vi "MDPtr Unpack WaveformArr.vi"(10 "error in (no error)":errorcluster, 11 "HexStrPtr":T1) -> (1 "String Attribute":string, 2 "error out":errorcluster, 3 "Waveforms":waveform(dbl)[](array[waveform]))   [LabVIEW 2017, in "MDPtr.lvlib"]
uses:
  MDPtr.lvlib
  MDPtr TypeDef/MDPtr.ctl
  MDPtr TypeDef/MDPtr SupportedDataTypeDef.ctl
  MDPtr TypeDef/MDPtr DataFrame-WaveformArr.ctl
  MDPtr TypeDef/MDPtr DataFrame-Common.ctl
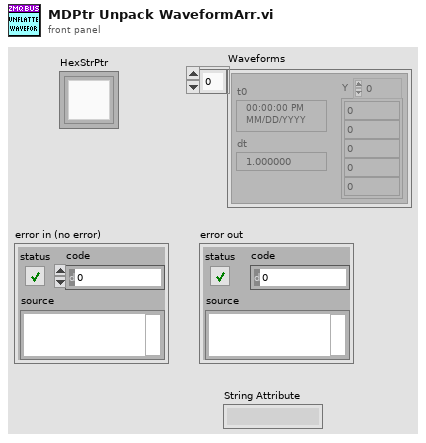
[diagram p1: front panel]
types:
  T1 = typedef "MDPtr.lvlib/MDPtr.ctl" = refnum<k1>
  T2 = typedef "MDPtr.lvlib/MDPtr SupportedDataTypeDef.ctl" = enum16{"<Invalid>", "<User 0>", "<User 1>", "<User 2>", "<User 3>", "<User 4>", "Memory", "Waveform", "Waveform Arr", "Double Arr", "String Arr"}
  T3 = typedef "MDPtr.lvlib/MDPtr DataFrame-WaveformArr.ctl" = cluster{"Common":T4, "DVR":refnum<data-value>}
  T4 = typedef "MDPtr.lvlib/MDPtr DataFrame-Common.ctl" = cluster{"Data Type":T2, "Copy Count":i32, "String Attribute":string}
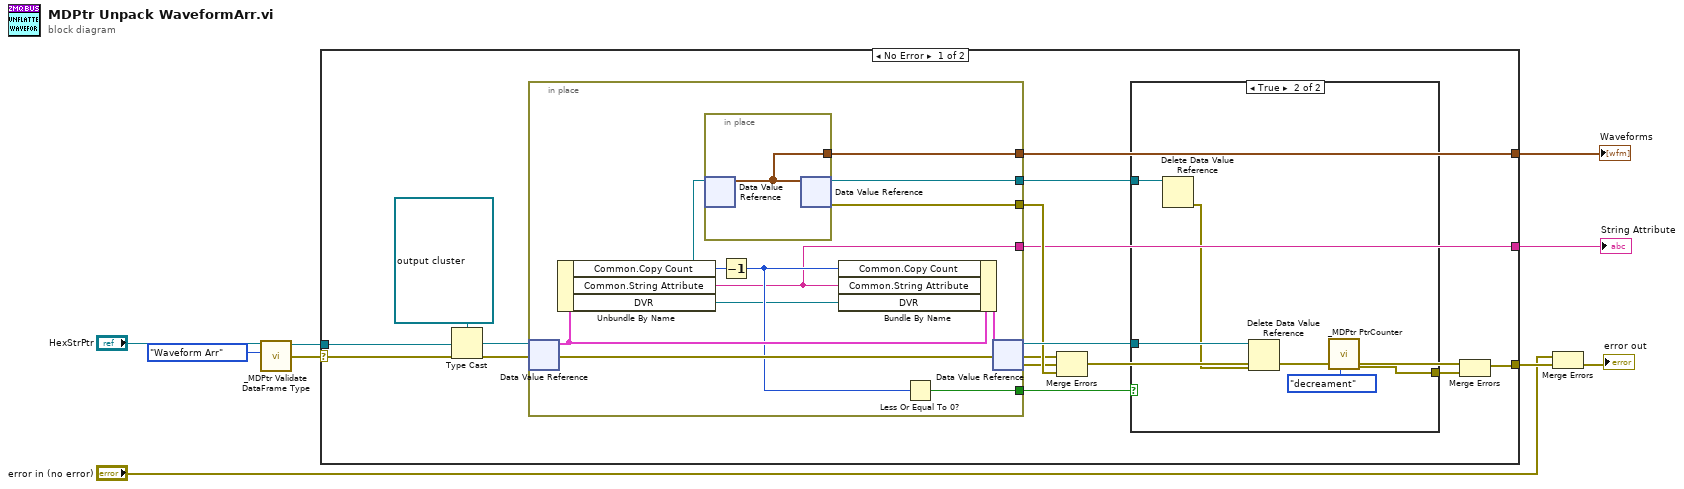
[diagram p0: block diagram]
diagram:
  n1 = call "_MDPtr Validate DataFrame Type.vi"("Data Type"=MDPtr_SupportedDataTypeDef."Waveform Arr", "data"="HexStrPtr") -> ("error out"=w2:errorcluster, "data (dup)"=w3:T1)  [unwired: 7 in]
  n2 = case shown="No Error" w2 {
    selector: w2 -> [w11 w41]
    tunnel: [w23 w41] -> w9
    tunnel: [w22 _] -> w7
    tunnel: w3 -> [w12 _]
    tunnel: [w10 _] -> w1
    frame No Error {
      n3 = Type Cast(type=refnum<data-value> refnum ("data value reference"), x=w12) -> (*(type *) &x=w18:refnum<data-value>)
      n4 = in-place {
        in-place-border: [w36] -> w22
        in-place-border: [w34] -> w19
        in-place-border: [w33] -> w21
        in-place-border: [w31] -> w16
        in-place-border: [w30] -> w10
        n5 = in-place-dvr #1(w18) -> (w39:T3)  [unwired: 1 out]
        n6 = Unbundle By Name(w39) -> ("Common.Copy Count"=w37:i32, "Common.String Attribute"=w30:string, "DVR"=w32:refnum<data-value>)
        n7 = in-place {
          in-place-border: [w40] -> w36
          n8 = in-place-dvr #2(w32) -> (w40:waveform(dbl)[])  [unwired: 1 out]
          n9 = in-place-dvr #2(w40) -> (w33:refnum<data-value>, w31:errorcluster)
        }
        n10 = Decrement(x=w37) -> (x-1=w35:i32)
        n11 = Bundle By Name(cluster=w39, "Common.Copy Count"=w35, "Common.String Attribute"=w30, "DVR"=w32) -> (w38:T3)
        n12 = Less Or Equal To 0?(x=w35) -> (x <= 0?=w34:bool)
        n13 = in-place-dvr #1(w38) -> (w20:refnum<data-value>, w15:errorcluster)
      }
      n14 = Merge Errors(w11, w15, w16) -> (w13:errorcluster)
      n15 = case shown="True" w19 {
        tunnel: w20 -> [_ w29]
        tunnel: w21 -> [_ w28]
        tunnel: [_ w24] -> w14
        frame False {
        }
        frame True {
          n16 = Delete Data Value Reference(data value reference=w28) -> (error out=w27:errorcluster)  [unwired: 1 in, 1 out]
          n17 = Delete Data Value Reference(data value reference=w29, error in=w27) -> (error out=w25:errorcluster)  [unwired: 1 out]
          n18 = call "_MDPtr PtrCounter.vi"("Oper(Get)"=enum16{"GET", "Increament", "decreament"}."decreament", "error in (no error)"=w25) -> ("error out"=w24:errorcluster)  [unwired: 8 in, 1 out]
        }
      }
      n19 = Merge Errors(w13, w14) -> (w23:errorcluster)
    }
    frame Error {
    }
  }
  "Waveforms" <- w7
  "String Attribute" <- w1
  n20 = Merge Errors("error in (no error)", w9) -> (→"error out":errorcluster)
